vi "Write DLL path_string.vi"(8 "error in (no error)":errorcluster, 10 "DLL path string":string, 11 "DelayLine in":refnum<class "DelayLine.lvclass">) -> (0 "error out":errorcluster, 3 "DelayLine out":refnum<class "DelayLine.lvclass">)   [LabVIEW 2018, in "DelayLine.lvclass"]
uses:
  DelayLine.lvclass
  DelayLine.lvclass/DelayLine.ctl
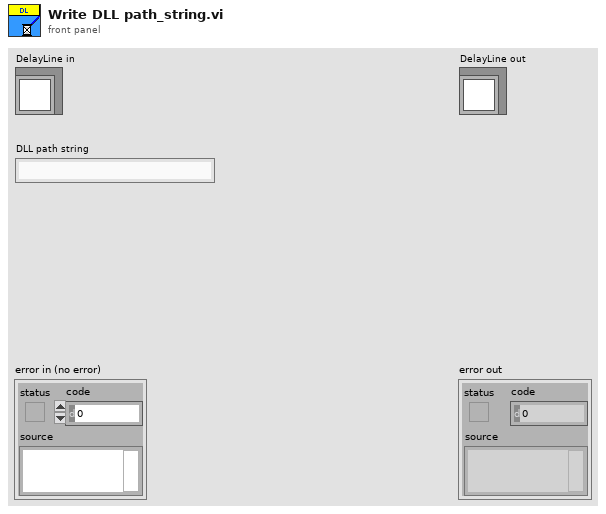
[diagram p1: front panel]
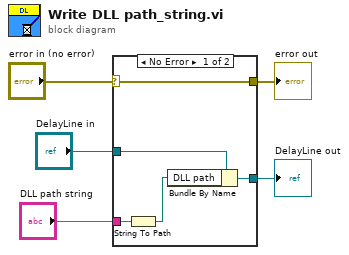
[diagram p0: block diagram]
diagram:
  n1 = case shown="No Error" "error in (no error)" {
    selector: "error in (no error)" -> [w10 w11]
    tunnel: [w10 w11] -> w4
    tunnel: [w8 w12] -> w2
    tunnel: "DelayLine in" -> [w9 w12]
    tunnel: "DLL path string" -> [w7 _]
    frame No Error {
      n2 = String To Path(string=w7) -> (path=w6:path)
      n3 = Bundle By Name(cluster=w9, "DLL path"=w6) -> (w8:refnum<class "DelayLine.lvclass">)
    }
    frame Error {
    }
  }
  "error out" <- w4
  "DelayLine out" <- w2
